vi "New Path Planner 2.vi"(11 "GIC Input":T1={"     Use ?\nOff       On"=[FALSE, TRUE, FALSE, TRUE], "Mode:"=FALSE, "Rx Prop Port"="", "Hokuyo Port"="COM7", "Tx Prop  Port"="COM6", "Compass Port"="", "GPS Port"="", "Num of WPs"=0, "WP Lats and Longs"={"WP Lats"=[], "WP Longs"=[]}, "Obst Lats and Longs"={"Obst Lats"=[], "Obst Longs"=[]}, "Parameters"=[], "GPS Data"=[], "Compass"=0.0, "LMS Vector"=[], "Vision Vector"=[], "Direction Cmd"=0.0, "Speed Cmd"=0.0, "WP Vector"=[], "WP Number"=0, "Extra"=0, "SW Map"=[], "Path Cluster"={"Path x node"=[], "Path y node"=[]}} {"Obst Lats and Longs"."Obst Longs" format="%#_8g"; "Obst Lats and Longs"."Obst Lats" format="%#_8g"}) -> (3 "GIC Output":T1={"     Use ?\nOff       On"=[FALSE, TRUE, FALSE, TRUE], "Mode:"=FALSE, "Rx Prop Port"="", "Hokuyo Port"="COM7", "Tx Prop  Port"="COM6", "Compass Port"="", "GPS Port"="", "Num of WPs"=0, "WP Lats and Longs"={"WP Lats"=[], "WP Longs"=[]}, "Obst Lats and Longs"={"Obst Lats"=[], "Obst Longs"=[]}, "Parameters"=[], "GPS Data"=[], "Compass"=0.0, "LMS Vector"=[], "Vision Vector"=[], "Direction Cmd"=0.0, "Speed Cmd"=0.0, "WP Vector"=[], "WP Number"=0, "Extra"=0, "SW Map"=[], "Path Cluster"={"Path x node"=[], "Path y node"=[]}} {"Obst Lats and Longs"."Obst Longs" format="%#_8g"; "Obst Lats and Longs"."Obst Lats" format="%#_8g"})   [LabVIEW 2014]
panel:
  # "New Path Planner 2"
  # "Input:"
  # "Output"
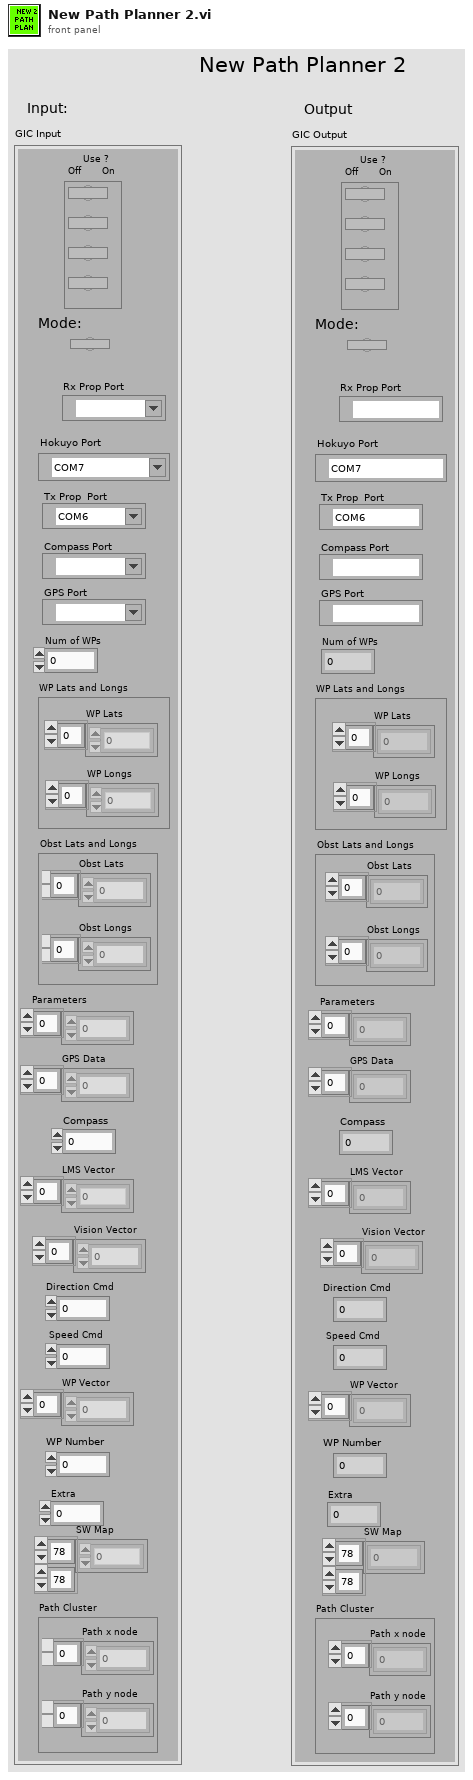
[diagram p1: front panel]
types:
  T1 = cluster{"     Use ?\nOff       On":bool[], "Mode:":bool, "Rx Prop Port":refnum<visa-resource-name>, "Hokuyo Port":refnum<visa-resource-name>, "Tx Prop  Port":refnum<visa-resource-name>, "Compass Port":refnum<visa-resource-name>, "GPS Port":refnum<visa-resource-name>, "Num of WPs":i16, "WP Lats and Longs":cluster{"WP Lats":dbl[], "WP Longs":dbl[]}, "Obst Lats and Longs":cluster{"Obst Lats":dbl[], "Obst Longs":dbl[]}, "Parameters":dbl[], "GPS Data":dbl[], "Compass":dbl, "LMS Vector":dbl[], "Vision Vector":dbl[], "Direction Cmd":dbl, "Speed Cmd":dbl, "WP Vector":dbl[], "WP Number":i32, "Extra":i16, "SW Map":i32[][], "Path Cluster":cluster{"Path x node":dbl[], "Path y node":dbl[]}}
  T2 = cluster{"     Use ?\nOff       On":bool[], "Mode:":bool, "Rx Prop Port":refnum<visa-resource-name>, "Hokuyo Port":refnum<visa-resource-name>, "Tx Prop Port":refnum<visa-resource-name>, "Compass Port":refnum<visa-resource-name>, "GPS Port":refnum<visa-resource-name>, "Num of WPs":i16, "WP Lats and Longs":cluster{"WP Lats":dbl[], "WP Longs":dbl[]}, "Obst Lats and Longs":cluster{"Obst Lats":dbl[], "Obst Longs":dbl[]}, "Parameters":dbl[], "GPS Data":dbl[], "Compass":dbl, "LMS Vector":dbl[], "Vision Vector":dbl[], "Direction Cmd":dbl, "Speed Cmd":dbl, "WP Vector":dbl[], "WP Number":i32, "Extra":i16, "SW Map":i32[][], "Path Cluster":cluster{"Path x node":dbl[], "Path y node":dbl[]}}
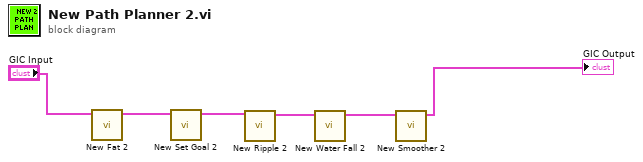
[diagram p0: block diagram]
diagram:
  n1 = call "New Fat 2.vi"("GIC Input"="GIC Input") -> ("GIC Output"=w5:T1)  [unwired: 10 in]
  n2 = call "New Set Goal 2.vi"("GIC Input"=w5) -> ("GIC Output"=w4:T1)  [unwired: 10 in]
  n3 = call "New Ripple 2.vi"("GIC Input"=w4) -> ("GIC Output"=w3:T1)  [unwired: 10 in]
  n4 = call "New Water Fall 2.vi"("GIC Input"=w3) -> ("GIC Output"=w2:T2)  [unwired: 10 in]
  n5 = call "New Smoother 2.vi"("GIC Input"=w2) -> ("GIC Output"=→"GIC Output":T1)  [unwired: 10 in]
